vi "Read Busy Flag and Address.vi"(6 "chip select  (1st chip)":enum16{"1st chip", "2nd chip"}(ring), 8 "error in (no error)":errorcluster, 11 "LCD in":refnum<class "Character LCD.lvclass">) -> (0 "error out":errorcluster, 1 "address":u8=97 format="%.0x", 2 "busy flag":bool, 3 "LCD out":refnum<class "Character LCD.lvclass">)   [LabVIEW 2017, in "HD44780 Host.lvlib"]
uses:
  HD44780 Host.lvlib
  Internal/LCD Class/Character LCD.lvclass
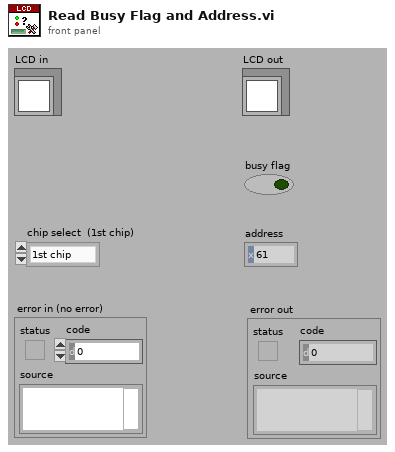
[diagram p1: front panel]
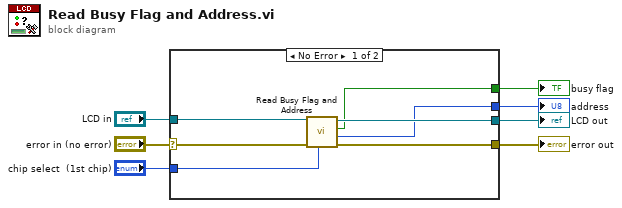
[diagram p0: block diagram]
diagram:
  n1 = case shown="No Error" "error in (no error)" {
    selector: "error in (no error)" -> [w10 w16]
    tunnel: [w11 w16] -> w7
    tunnel: "chip select  (1st chip)" -> [w14 _]
    tunnel: "LCD in" -> [w13 w15]
    tunnel: [w12 w15] -> w3
    tunnel: [w9 _] -> w2
    tunnel: [w8 _] -> w1
    frame No Error {
      n2 = call-dynamic "Read Busy Flag and Address.vi"("chip select  (1st chip)"=w14, "error in (no error)"=w10, "Character LCD in"=w13) -> ("error out"=w11:errorcluster, "address"=w9:u8, "busy flag"=w8:bool, "Character LCD out"=w12:refnum<class "Character LCD.lvclass">)  [unwired: 5 in]
    }
    frame Error {
    }
  }
  "error out" <- w7
  "LCD out" <- w3
  "busy flag" <- w1
  "address" <- w2
